vi "7.3 - Has Mission Def.vi"   [LabVIEW 2010]
uses:
  7.6 - GPS Waypoint Def.ctl
  6-OCU Neurons/MDF Array LatLong.ctl
  6-OCU Neurons/MDF LatLong.ctl
  7.0-Global.vi
types:
  T1 = typedef "7.6 - GPS Waypoint Def.ctl" = cluster{"GPS Waypoint Center (Lat, Long)":dbl[], "5.1.1 MDF GPS":T2}
  T2 = typedef "MDF Array LatLong.ctl" = T3[]
  T3 = typedef "MDF LatLong.ctl" = cluster{"Waypoint #":dbl, "Latitude (waypoint)":ext, "Longitude  (waypoint)":ext}
  T4 = cluster{"GPS Waypoint Center (Lat, Long)":bool[], "5.1.1 MDF GPS":cluster{"Waypoint #":bool, "Latitude (waypoint)":bool, "Longitude  (waypoint)":bool}[]}
  T5 = cluster{"Waypoint #":bool, "Latitude (waypoint)":bool, "Longitude  (waypoint)":bool}[]
  T6 = cluster{"Waypoint #":bool, "Latitude (waypoint)":bool, "Longitude  (waypoint)":bool}
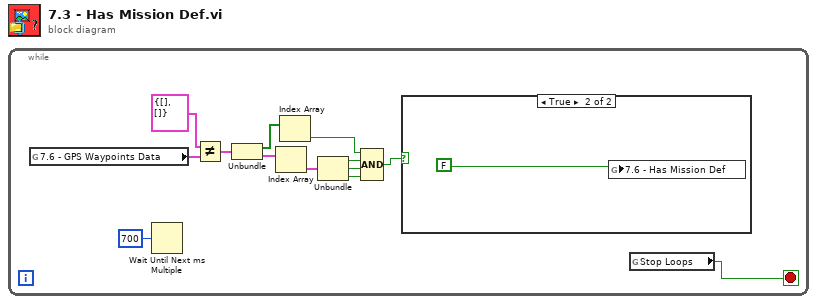
[diagram p0: block diagram]
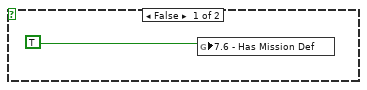
[diagram p2: hidden frame]
diagram:
  n1 = while {
    stop <- w2 stop-if-true
    n2 = global read "7.0-Global.vi" "7.6 - GPS Waypoints Data"() -> (w4:T1)
    n3 = Wait Until Next ms Multiple(millisecond multiple=u32 700) -> ()  [unwired: 1 out]
    n4 = Not Equal?(x=T1 {"GPS Waypoint Center (Lat, Long)"=[], "5.1.1 MDF GPS"=[]} ("7.6 - GPS Waypoints Data 2"), y=w4) -> (x != y?=w5:T4)
    n5 = Unbundle(w5) -> ("GPS Waypoint Center (Lat, Long)"=w11:bool[], "5.1.1 MDF GPS"=w6:T5)
    n6 = Index Array(array=w6) -> (element=w7:T6)  [unwired: 1 in]
    n7 = Index Array(array=w11) -> (element=w12:bool)  [unwired: 1 in]
    n8 = Unbundle(w7) -> ("Waypoint #"=w8:bool, "Latitude (waypoint)"=w9:bool, "Longitude  (waypoint)"=w10:bool)
    n9 = Compound Arithmetic op=AND(w12, w8, w9, w10) -> (w13:bool)
    n10 = case shown="True" w13 {
      frame False {
        n11 = global write "7.0-Global.vi" "7.6 - Has Mission Def"(TRUE ("Has Mission Def")) -> ()
      }
      frame True {
        n12 = global write "7.0-Global.vi" "7.6 - Has Mission Def"(FALSE ("Has Mission Def")) -> ()
      }
    }
    n13 = global read "7.0-Global.vi" "Stop Loops"() -> (w2:bool)
  }
